vi "Post-Install Custom Action.vi"(10 "Variant":variant) -> (0 "error out":errorcluster)   [LabVIEW 2021]
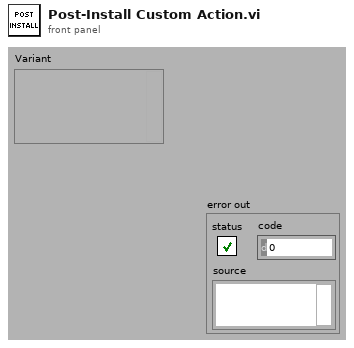
[diagram p1: front panel]
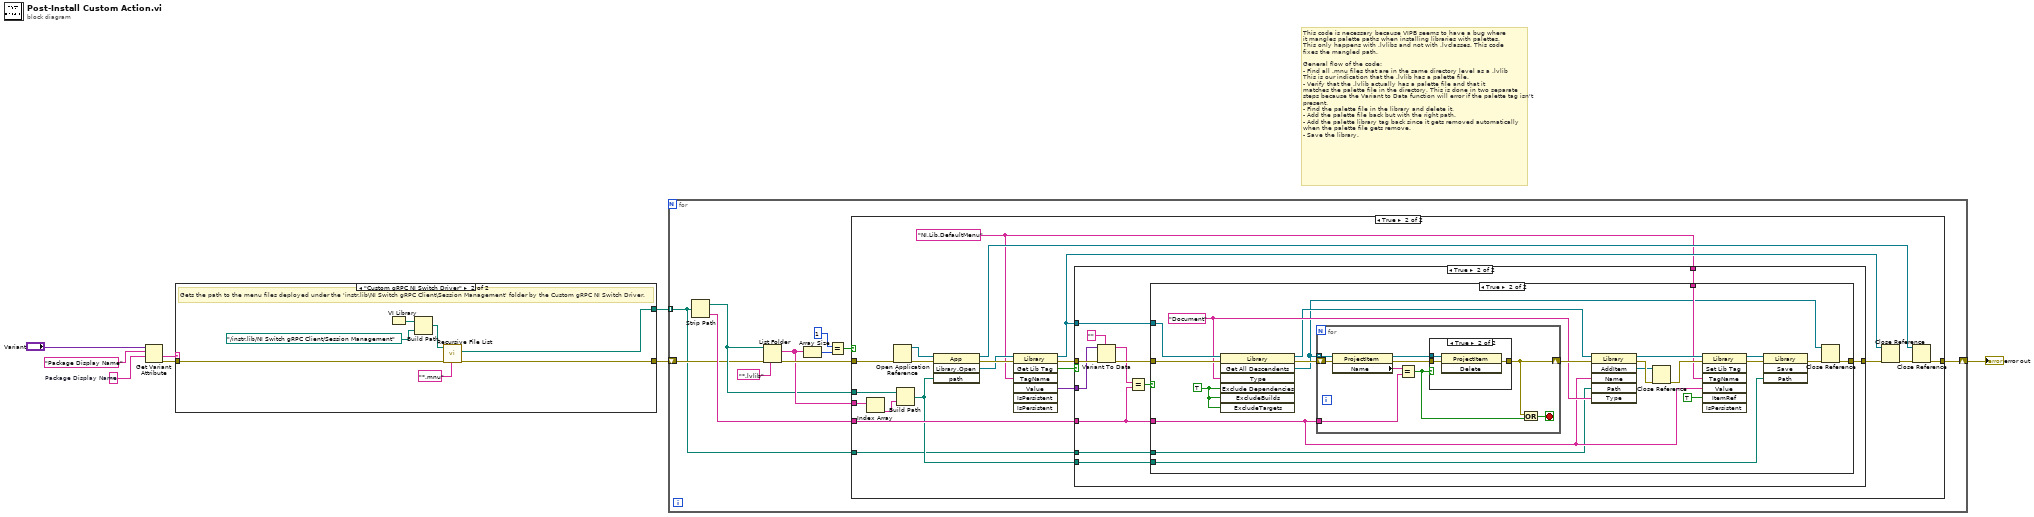
[diagram p0: block diagram]
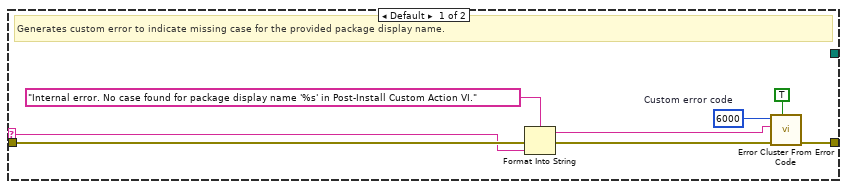
[diagram p6: hidden frame]
diagram:
  w7 = ""  # Package Display Name
  # "This code is necessary because VIPB seems to have a bug where\nit mangles palette paths when installing libraries with palettes.\nThis only happens with .lvlibs and not with .lvclasses. This code\nfixes the mangled path.\n\nGeneral flow of the code:\n- Find all .mnu files that are in the same directory level as a .lvlib\nThis is our indication that the .lvlib has a palette file.\n- Verify that the .lvlib actually has a palette file and that it\nmatches the palette file in the directory. This is done in two separate\nsteps because the Variant to Data function will error if the palette tag isn't\npresent.\n- Find the palette file in the library and delete it.\n- Add the palette file back but with the right path.\n- Add the palette library tag back since it gets removed automatically\nwhen the palette file gets remove.\n- Save the library."
  n1 = Get Variant Attribute(Variant="Variant", name="Package Display Name", default value (empty Variant)=w7) -> (value=w2:string, error out=w1:errorcluster)  [unwired: 1 in, 2 out]
  n2 = case shown="\"Custom gRPC NI Switch Driver\"" w2 {
    selector: w2 -> [w13 _]
    tunnel: [_ w18] -> w3
    tunnel: [w16 w19] -> w4
    tunnel: w1 -> [w14 w17]
    frame Default {
      w11 = 6000  # Custom error code
      # "Generates custom error to indicate missing case for the provided package display name."
      n3 = Format Into String(format string="Internal error. No case found for package display name '%s' in Post-Install Custom Action VI.", error in=w14, w13) -> (resulting string=w12:string, error out=w15:errorcluster)  [unwired: 1 in]
      n4 = call <vilib>:"Error Cluster From Error Code.vi"("show call chain? (False)"=TRUE, "error in (no error)"=w15, "error message (\"\")"=w12, "error code (0)"=w11) -> ("error out"=w16:errorcluster)  [unwired: 5 in]
    }
    frame "Custom gRPC NI Switch Driver" {
      # "Gets the path to the menu files deployed under the 'instr.lib\\NI Switch gRPC Client\\Session Management' folder by the Custom gRPC NI Switch Driver."
      n5 = VI Library() -> (path=w22:path)
      n6 = Build Path(base path=w22, name or relative path=path "../instr.lib/NI Switch gRPC Client/Session Management") -> (appended path=w23:path)
      n7 = call <vilib>:"Recursive File List.vi"("pattern"="*.mnu", "error in (no error)"=w17, "Folder Path"=w23) -> ("error out"=w19:errorcluster, "All Files in Dir"=w18:path[])  [unwired: 4 in, 3 out]
    }
  }
  n8 = for {
    shift-right: [w26] -> w6
    shift-left: w4 -> [w25]
    tunnel: w3 -> [w24] mode=indexing
    n9 = Strip Path(path=w24) -> (stripped path=w28:path, name=w32:string)
    n10 = List Folder(path=w28, pattern="*.lvlib", error in=w25) -> (filenames=w30:string[], error out=w31:errorcluster)  [unwired: 1 in, 2 out]
    n11 = Array Size(array=w30) -> (size(s)=w34:i32)
    n12 = Equal?(x=1, y=w34) -> (x = y?=w33:bool)
    n13 = case shown="True" w33 {
      tunnel: w31 -> [w35 w52]
      tunnel: w30 -> [_ w55]
      tunnel: w32 -> [_ w47]
      tunnel: w28 -> [_ w43]
      tunnel: [w35 w37] -> w26
      tunnel: w24 -> [_ w36]
      frame False {
      }
      frame True {
        w39 = "NI.Lib.DefaultMenu" ("Tag Name")
        n14 = Index Array(array=w55) -> (element=w42:string)  [unwired: 1 in]
        n15 = Open Application Reference(8:w52) -> (0:w54:errorcluster, 3:w53:refnum<vi>)  [unwired: 3 in]
        n16 = Build Path(base path=w43, name or relative path=w42) -> (appended path=w41:path)
        n17 = invoke class="App" method="Library.Open"(reference=w53, error in=w54, "path"=w41) -> (reference out=w44:refnum<vi>, error out=w51:errorcluster, "Open Library"=w48:refnum<vi>)  [unwired: 1 in, 1 out]
        n18 = invoke class="Library" method="Get Lib Tag"(reference=w48, error in=w51, "TagName"=w39) -> (reference out=w45:refnum<vi>, error out=w49:errorcluster, "GetTag"=w40:bool, "Value"=w50:variant)  [unwired: 4 in, 3 out]
        n19 = case shown="True" w40 {
          tunnel: w50 -> [_ w64]
          tunnel: w49 -> [w56 w65]
          tunnel: [w56 w68] -> w46
          tunnel: w45 -> [_ w67]
          tunnel: w41 -> [_ w66]
          tunnel: w47 -> [_ w60]
          tunnel: w39 -> [_ w58]
          tunnel: w36 -> [_ w57]
          frame False {
          }
          frame True {
            n20 = Variant To Data(error in=w65, type="", Variant=w64) -> (data=w61:string, error out=w63:errorcluster)
            n21 = Equal?(x=w61, y=w60) -> (x = y?=w59:bool)
            n22 = case shown="True" w59 {
              tunnel: [w69 w79] -> w68
              tunnel: w67 -> [_ w90]
              tunnel: w66 -> [_ w85]
              tunnel: w63 -> [w69 w84]
              tunnel: w60 -> [_ w71]
              tunnel: w58 -> [_ w76]
              tunnel: w57 -> [_ w70]
              frame False {
              }
              frame True {
                w78 = "Document" ("Type")
                w74 = TRUE ("ExcludeDependencies")
                n23 = invoke class="Library" method="Get All Descendents"(reference=w90, error in=w84, "Type"=w78, "Exclude Dependencies"=w74, "ExcludeBuilds"=w74, "ExcludeTargets"=w74) -> (reference out=w73:refnum<vi>, error out=w89:errorcluster, "All Descendents"=w72:refnum<vi>[])  [unwired: 1 in, 4 out]
                n24 = for {
                  tunnel: w72 -> [w99] mode=indexing
                  shift-right: [w93] -> w88
                  shift-left: w89 -> [w95]
                  tunnel: w71 -> [w94]
                  stop <- w91 stop-if-true
                  n25 = property class="ProjectItem"(reference=w99, error in=w95) -> (reference out=w97:refnum<vi>, error out=w96:errorcluster, "Name"=w98:string)
                  n26 = Equal?(x=w98, y=w94) -> (x = y?=w92:bool)
                  n27 = case shown="True" w92 {
                    tunnel: w97 -> [_ w103]
                    tunnel: w96 -> [w100 w101]
                    tunnel: [w100 w102] -> w93
                    frame False {
                    }
                    frame True {
                      n28 = invoke class="ProjectItem" method="Delete"(reference=w103, error in=w101) -> (error out=w102:errorcluster)  [unwired: 1 in, 2 out]
                    }
                  }
                  n29 = Or(x=w93, y=w92) -> (x .or. y?=w91:bool)
                }
                n30 = invoke class="Library" method="AddItem"(reference=w73, error in=w88, "Name"=w71, "Path"=w70, "Type"=w78) -> (reference out=w77:refnum<vi>, error out=w82:errorcluster, "AddItem"=w81:refnum<vi>)  [unwired: 1 in, 3 out]
                n31 = Close Reference(reference=w81, error in (no error)=w82) -> (error out=w80:errorcluster)
                n32 = invoke class="Library" method="Set Lib Tag"(reference=w77, error in=w80, "TagName"=w76, "Value"=w71, "ItemRef"=TRUE ("Is Persistent")) -> (reference out=w87:refnum<vi>, error out=w86:errorcluster)  [unwired: 2 in, 5 out]
                n33 = invoke class="Library" method="Save"(reference=w87, error in=w86, "Path"=w85) -> (error out=w83:errorcluster)  [unwired: 1 in, 3 out]
                n34 = Close Reference(reference=w72, error in (no error)=w83) -> (error out=w79:errorcluster)
              }
            }
          }
        }
        n35 = Close Reference(reference=w45, error in (no error)=w46) -> (error out=w38:errorcluster)
        n36 = Close Reference(reference=w44, error in (no error)=w38) -> (error out=w37:errorcluster)
      }
    }
  }
  "error out" <- w6
